vi "Array-Concat Columns (DBL).vi"(4 "Array 2":dbl[][](array[numeric]), 5 "Array 1":dbl[][](array[numeric])) -> (1 "concatenated array":dbl[][](array[numeric]))   [LabVIEW 2020]
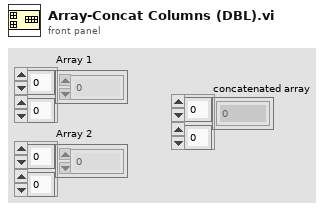
[diagram p1: front panel]
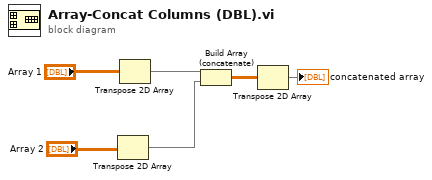
[diagram p0: block diagram]
diagram:
  n1 = Transpose 2D Array(2D array="Array 2") -> (transposed array=w3:dbl[][])
  n2 = Transpose 2D Array(2D array="Array 1") -> (transposed array=w4:dbl[][])
  n3 = Build Array (concatenate)(w4, w3) -> (w2:dbl[][])
  n4 = Transpose 2D Array(2D array=w2) -> (transposed array=→"concatenated array":dbl[][])
